vi "baselines2.vi"() -> ()   [LabVIEW 2009]
uses:
  <vilib>/Analysis/baseanly.llb/Unimode.vi
  <vilib>/Utility/file.llb/Read From Spreadsheet File (DBL).vi
  <vilib>/Analysis/NI_AALBase.lvlib
panel:
  in  "index (row)":i32
  in  "intervals":i32=100
  out "subarray":dbl[][](graph)
  out "Histogram Graph":T1(graph)
  in  "number of rows (all:-1)":i32=300
  in  "file path (dialog if empty)":path
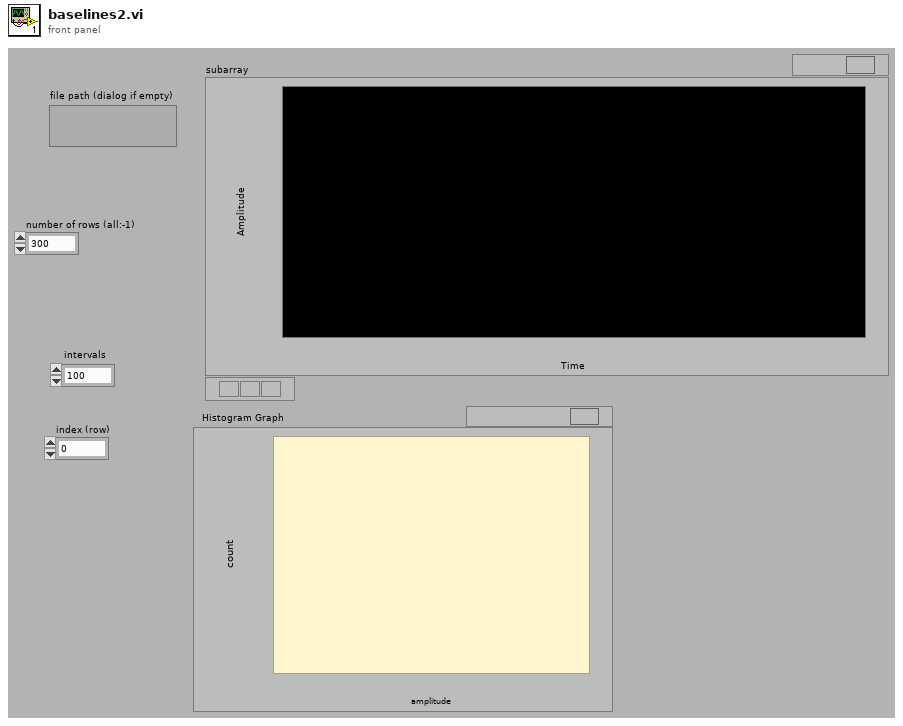
[diagram p1: front panel]
types:
  T1 = cluster{"X Values":dbl[], "Histogram: h(x)":i32[]}
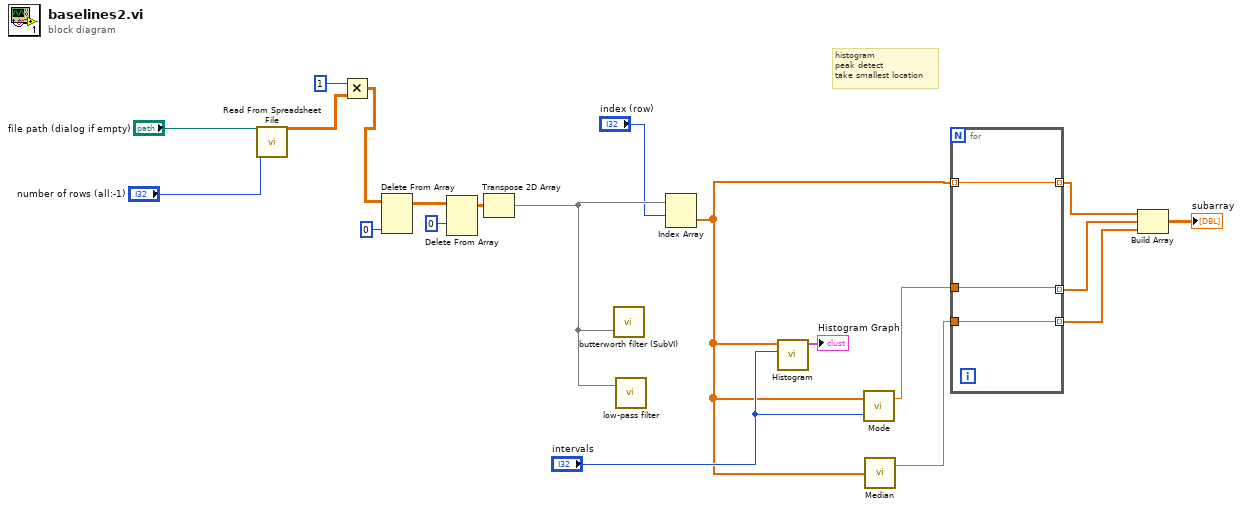
[diagram p0: block diagram]
diagram:
  # "histogram\npeak detect\ntake smallest location"
  n1 = call-poly <vilib>:"Read From Spreadsheet File.vi"("number of rows (all:-1)"="number of rows (all:-1)", "file path (dialog if empty)"="file path (dialog if empty)") -> ("all rows"=w13:dbl[][])  [unwired: 5 in, 4 out]
  n2 = Multiply(x=1 ("disabled index (col)"), y=w13) -> (x*y=w12:dbl[][])
  n3 = Delete From Array(array=w12, index (col)=0 ("disabled index (col)")) -> (array with subset deleted=w16:dbl[][])  [unwired: 2 in, 1 out]
  n4 = Delete From Array(array=w16, index (row)=0 ("disabled index (col)")) -> (array with subset deleted=w15:dbl[][])  [unwired: 2 in, 1 out]
  n5 = Transpose 2D Array(2D array=w15) -> (transposed array=w11:dbl[][])
  n6 = call "butterworth filter (SubVI).vi"("Array 2"=w11) -> ()  [unwired: 1 in, 1 out]
  n7 = call "low-pass filter.vi"("Array 2"=w11) -> ()  [unwired: 1 in, 1 out]
  n8 = Index Array(array=w11, index (row)="index (row)") -> (element=w8:dbl[])  [unwired: 1 in]
  n9 = call <vilib>:"Histogram.vi"("intervals"="intervals", "X"=w8) -> ("Histogram Graph"=→"Histogram Graph":T1)  [unwired: 6 in, 3 out]
  n10 = call-poly <vilib>:"Mode.vi"("intervals"="intervals", "X"=w8) -> ("mode"=w7:dbl)  [unwired: 1 out]
  n11 = call <vilib>:"Median.vi"("X"=w8) -> ("median"=w6:dbl)  [unwired: 1 out]
  n12 = for {
    tunnel: w8 -> [w21] mode=indexing
    tunnel: w7 -> [w23]
    tunnel: w6 -> [w22]
    tunnel: [w23] -> w4 mode=indexing
    tunnel: [w22] -> w3 mode=indexing
    tunnel: [w21] -> w5 mode=indexing
  }
  n13 = Build Array(w5, w4, w3) -> (→"subarray":dbl[][])
